vi "Test mysql queries with class.vi"() -> ()   [LabVIEW 2020, in "mysql-queries.lvlib" / "mysql-queries.lvclass"]
uses:
  mysql-queries.lvclass
  externals/mysql/Source/mysql.net/mysql.lvclass
panel:
  out "x = y?":bool
  out "Result":string
  out "error out":errorcluster
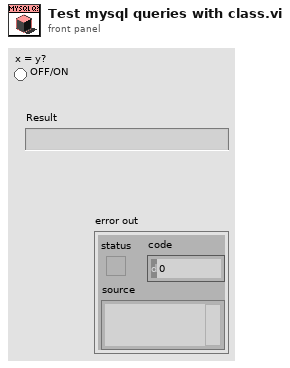
[diagram p1: front panel]
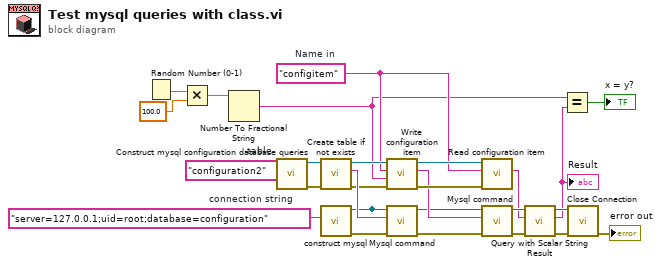
[diagram p0: block diagram]
diagram:
  w6 = "configitem"  # Name in
  w14 = "configuration2"  # table
  w23 = "server=127.0.0.1;uid=root;database=configuration"  # connection string
  n1 = Random Number (0-1)() -> (number: 0 to 1=w9:dbl)
  n2 = Multiply(x=w9, y=100.0) -> (x*y=w7:dbl)
  n3 = Number To Fractional String(number=w7) -> (F-format string=w5:string)  [unwired: 3 in]
  n4 = call "Construct mysql configuration database queries.vi"("table"=w14) -> ("error out"=w15:errorcluster, "mysql-configdb-queries out"=w10:refnum<class "mysql-queries.lvclass">)  [unwired: 9 in]
  n5 = call-dynamic "Create table if not exists.vi"("error in (no error)"=w15, "IConfigDBQueries in"=w10) -> ("error out"=w13:errorcluster, "Query out"=w16:string)  [unwired: 8 in]
  n6 = call "construct mysql.vi"("Connection string"=w23) -> ("error out"=w18:errorcluster, "mysql out"=w2:refnum<class "mysql.lvclass">)  [unwired: 9 in]
  n7 = call-dynamic "Write configuration item.vi"("error in (no error)"=w13, "Value"=w5, "Name in"=w6, "IConfigDBQueries in"=w10) -> ("error out"=w12:errorcluster, "Query"=w11:string)  [unwired: 6 in]
  n8 = call "Mysql command.vi"("error in (no error)"=w18, "Query string"=w16, "mysql in"=w2) -> ("error out"=w17:errorcluster)  [unwired: 7 in, 1 out]
  n9 = call-dynamic "Read configuration item.vi"("error in (no error)"=w12, "configuration item"=w6, "IConfigDBQueries in"=w10) -> ("result"=w1:string)  [unwired: 7 in, 1 out]
  n10 = call "Mysql command.vi"("error in (no error)"=w17, "Query string"=w11, "mysql in"=w2) -> ("error out"=w22:errorcluster)  [unwired: 7 in, 1 out]
  n11 = call-dynamic "Query with Scalar String Result.vi"("error in (no error)"=w22, "Query string"=w1, "mysql in"=w2) -> ("error out"=w20:errorcluster, "Result"=w4:string, "mysql out"=w21:refnum<class "mysql.lvclass">)  [unwired: 6 in]
  "Result" <- w4
  n12 = Equal?(x=w5, y=w4) -> (x = y?=→"x = y?":bool)
  n13 = call-dynamic "Close Connection.vi"("error in (no error)"=w20, "mysql in"=w21) -> ("error out"=→"error out":errorcluster)  [unwired: 8 in, 1 out]
